vi "Check Send HB.vi"(7 "UDP":refnum<k16>, 11 "Subscription Loop Data in":T1) -> (3 "Subscription Loop Data":T1)   [LabVIEW 2020, in "Vecto.lvlib" / "RemoteDataService.lvclass"]
uses:
  RemoteDataService.lvclass
  Subscription Loop Data.ctl
  Subscription Group Info.ctl
  Group/Group.lvclass
  SubscribedDataHandler/SubscribedDataHandler.lvclass
  proto/UdpPayload/Data.ctl
  RemoteDataService.lvclass/RemoteDataService.ctl
  proto/UdpPayload/UdpPayload.lvlib
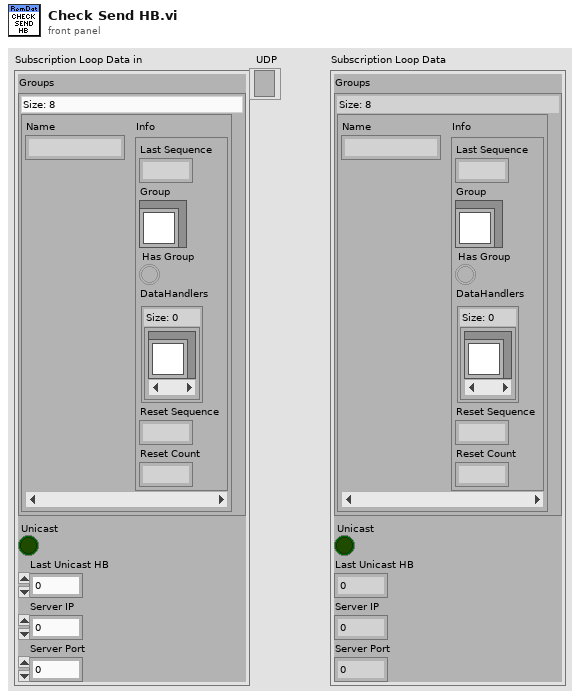
[diagram p1: front panel]
types:
  T1 = typedef "Vecto.lvlib/RemoteDataService.lvclass/Subscription Loop Data.ctl" = cluster{"Groups":map{string, T2}, "Unicast":bool, "Last Unicast HB":dbl, "Server IP":u32, "Server Port":u16}
  T2 = typedef "Vecto.lvlib/RemoteDataService.lvclass/Subscription Group Info.ctl" = cluster{"Last Sequence":u32, "Group":refnum<class "Group.lvclass">, "Has Group":bool, "DataHandlers":set{refnum<class "SubscribedDataHandler.lvclass">}, "Reset Sequence":u32, "Reset Count":u32}
  T3 = typedef "UdpPayload.lvlib/Data.ctl" = cluster{"source_id":u32, "sequence":u32, "timestamp":i64, "type":string, "payload":u8[]}
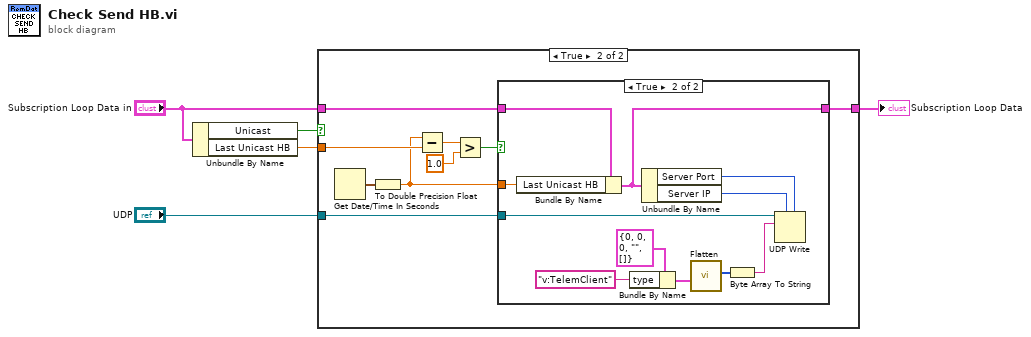
[diagram p0: block diagram]
diagram:
  n1 = Unbundle By Name("Subscription Loop Data in") -> ("Unicast"=w4:bool, "Last Unicast HB"=w2:dbl)
  n2 = case shown="True" w4 {
    tunnel: "Subscription Loop Data in" -> [w6 w9]
    tunnel: [w6 w8] -> w3
    tunnel: w2 -> [_ w14]
    tunnel: "UDP" -> [_ w7]
    frame False {
    }
    frame True {
      n3 = Get Date/Time In Seconds() -> (seconds since 1Jan1904=w15:timestamp)
      n4 = To Double Precision Float(number=w15) -> (double precision float=w10:dbl)
      n5 = Subtract(x=w10, y=w14) -> (x-y=w13:dbl)
      n6 = Greater?(x=w13, y=1.0) -> (0:w11:bool)
      n7 = case shown="True" w11 {
        tunnel: w10 -> [_ w22]
        tunnel: w9 -> [w16 w23]
        tunnel: [w16 w19] -> w8
        tunnel: w7 -> [_ w21]
        frame False {
        }
        frame True {
          n8 = Bundle By Name(cluster=w23, "Last Unicast HB"=w22) -> (w19:T1)
          n9 = Bundle By Name(cluster=T3 {"source_id"=0, "sequence"=0, "timestamp"=0, "type"="", "payload"=[]} ("Data"), "type"="v:TelemClient") -> (w26:T3)
          n10 = Unbundle By Name(w19) -> ("Server Port"=w17:u16, "Server IP"=w18:u32)
          n11 = call "Flatten.vi"("Data"=w26) -> ("Buffer"=w24:u8[])  [unwired: 9 in, 1 out]
          n12 = Byte Array To String(unsigned byte array=w24) -> (string=w20:string)
          n13 = UDP Write(address=w18, port or service name=w17, connection ID=w21, data in=w20) -> ()  [unwired: 2 in, 2 out]
        }
      }
    }
  }
  "Subscription Loop Data" <- w3
